vi "Send Launch Measurements Message.vi"(4 "Continuous Run":bool, 6 "Show FP?":bool, 7 "Iterations":i32, 8 "error in (no error)":errorcluster, 9 "Device Names":string[](array[string]), 10 "Measurement Name":string, 11 "Self Enqueuer In":refnum<class "Message Enqueuer.lvclass">) -> (0 "error out":errorcluster, 3 "Self Enqueuer Out":refnum<class "Message Enqueuer.lvclass">)   [LabVIEW 2017, in "Controller Actor.lvlib" / "Launch Measurements Message.lvclass"]
uses:
  Launch Measurements Message.lvclass
  <vilib>/ActorFramework/Message Enqueuer/Message Enqueuer.lvclass
  C:/Program Files (x86)/National Instruments/LabVIEW 2017/vi.lib/ActorFramework/Message/Message.lvclass
  Launch Measurements Message.lvclass/Launch Measurements Message.ctl
  <vilib>/ActorFramework/Message Enqueuer/Message Enqueuer.lvclass/Message Enqueuer.ctl
  <vilib>/ActorFramework/Message Priority Queue/Priority Enqueue.vi
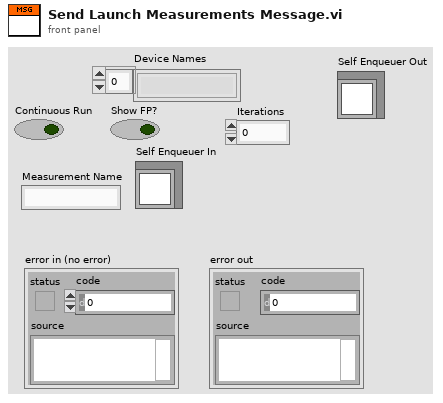
[diagram p1: front panel]
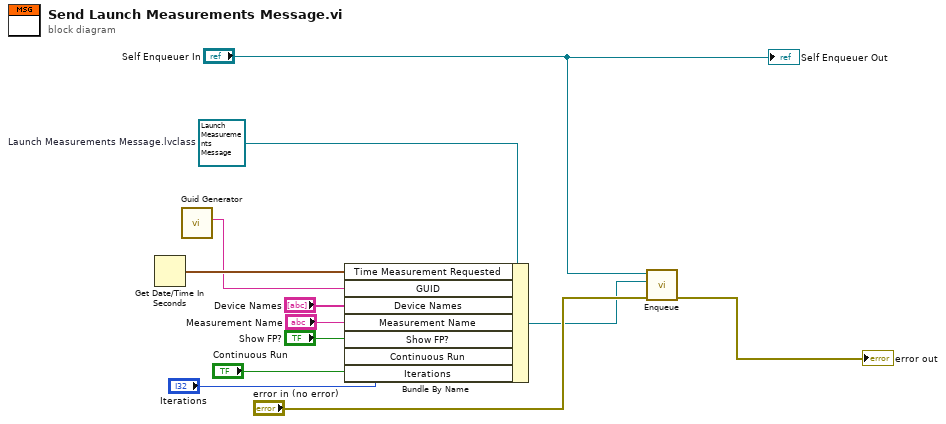
[diagram p0: block diagram]
diagram:
  w7 = refnum<class "Launch Measurements Message.lvclass"> refnum  # Launch Measurements Message.lvclass
  n1 = Get Date/Time In Seconds() -> (seconds since 1Jan1904=w8:timestamp)
  n2 = call <vilib>:"Guid Generator.vi"() -> ("GUID"=w6:string)  [unwired: 10 in, 1 out]
  n3 = Bundle By Name(cluster=w7, "Time Measurement Requested"=w8, "GUID"=w6, "Device Names"="Device Names", "Measurement Name"="Measurement Name", "Show FP?"="Show FP?", "Continuous Run"="Continuous Run", "Iterations"="Iterations") -> (w9:refnum<class "Launch Measurements Message.lvclass">)
  n4 = call <vilib>:"Enqueue.vi"("error in (no error)"="error in (no error)", "Message"=w9, "Message Enqueuer in"="Self Enqueuer In") -> ("error out"=→"error out":errorcluster)  [unwired: 7 in, 1 out]
  "Self Enqueuer Out" <- "Self Enqueuer In"
